vi "Read Power time.vi"(8 "error in (no error)":errorcluster, 11 "SciShutt in":refnum<class "SciShutt.lvclass">) -> (0 "error out":errorcluster, 2 "Power time":dbl, 3 "SciShutt out":refnum<class "SciShutt.lvclass">)   [LabVIEW 2016, in "SciShutt.lvclass"]
uses:
  SciShutt.lvclass
  SciShutt.lvclass/SciShutt.ctl
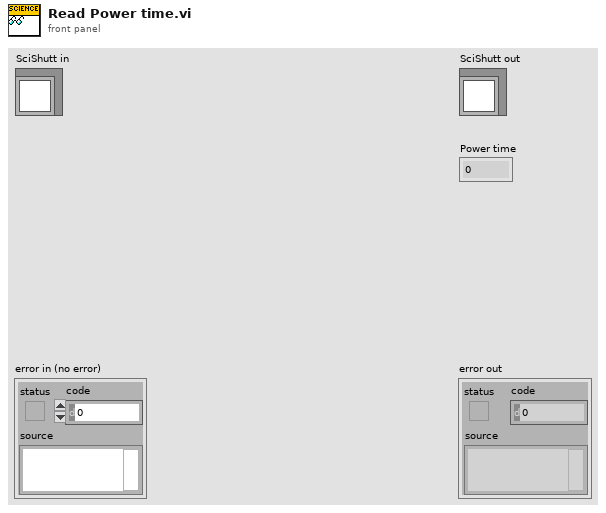
[diagram p1: front panel]
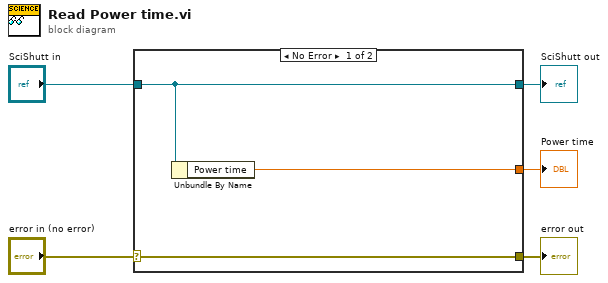
[diagram p0: block diagram]
diagram:
  n1 = case shown="No Error" "error in (no error)" {
    selector: "error in (no error)" -> [w8 w9]
    tunnel: [w8 w9] -> w4
    tunnel: [w7 w10] -> w2
    tunnel: "SciShutt in" -> [w7 w10]
    tunnel: [w6 _] -> w1
    frame No Error {
      n2 = Unbundle By Name(w7) -> ("Power time"=w6:dbl)
    }
    frame Error {
    }
  }
  "error out" <- w4
  "SciShutt out" <- w2
  "Power time" <- w1
